vi "Help Window 3.1.vi"() -> ()   [LabVIEW 2020]
panel:
  in  "Okay":bool
  # "The event selection menu will open from here. You will also select sensors to analyze.\n\nIf the file you have chosen does not have event annotations, this button will change and prompt you to find and open the associated XML file."
  # "Messages will appear here to help guide you."
  # "Click here to open the file of an HRM exam."
  # "This will open SPARC analysis for the event you select. The only user input needed is selectecting the bounds of the event so the program can easily find what its looking for."
  # "This will open NMD analysis for the event you select. The only user input needed is selectecting the bounds of the event so the program can easily find what its looking for."
  # "Clicking this will allow you to select a folder. From that folder, this will find all the available segments and run them automatically through the SPARC analysis. Note, this will only work if the segments are in a folder named \"Segments\"."
  # "To change the SPARC analysis setting (cut-off frequency, amplitude threshold, and pad level), click here."
  # "This will prompt you to select a folder of subjects. It will then find all of the smoothness results and compile the means of the data into a text file."
  # "Opens a menu consisting of options for different figures & images you can create/save."
  # "You clicked this to get here."
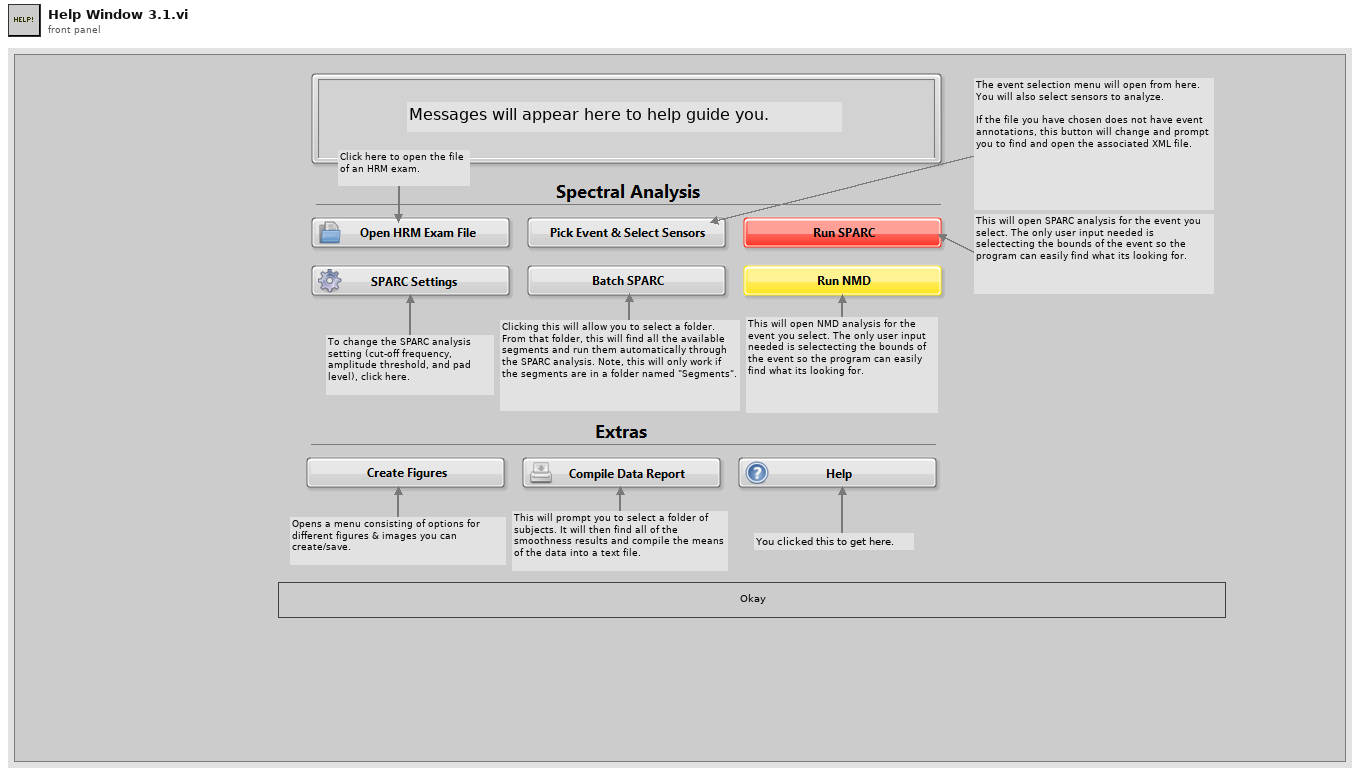
[diagram p1: front panel]
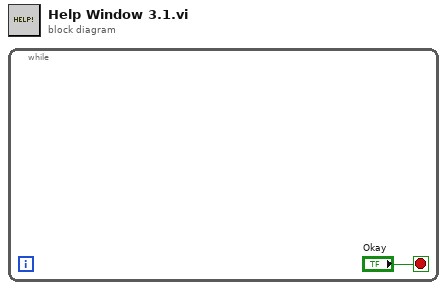
[diagram p0: block diagram]
diagram:
  n1 = while {
    stop <- "Okay" stop-if-true
  }
